vi "Init SVs.vi"(5 "error in":errorcluster) -> (19 "error out":errorcluster)   [LabVIEW 2015, in "cCRDS.lvclass"]
uses:
  cCRDS.lvclass
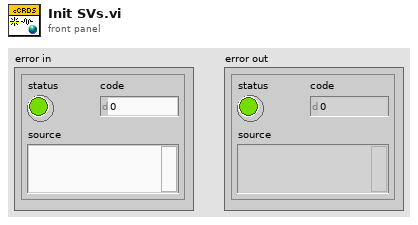
[diagram p1: front panel]
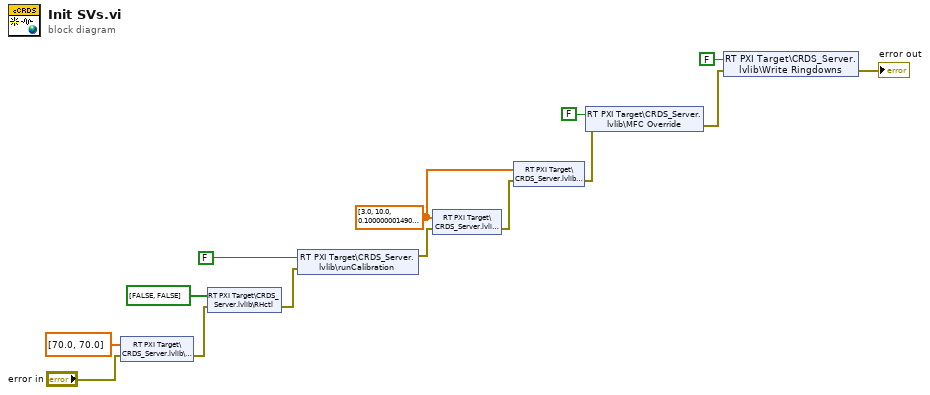
[diagram p0: block diagram]
diagram:
  w4 = sgl[] [3.0, 10.0, 0.1] ("Med")
  n1 = shared-variable "RT PXI Target\\CRDS_Server.lvlib\\RHsp"(sgl[] [70.0, 70.0] ("RHsp"), error in="error in") -> (error out=w13:errorcluster)
  n2 = shared-variable "RT PXI Target\\CRDS_Server.lvlib\\RHctl"(bool[] [FALSE, FALSE] ("RHctl"), error in=w13) -> (error out=w10:errorcluster)
  n3 = shared-variable "RT PXI Target\\CRDS_Server.lvlib\\runCalibration"(FALSE ("runCalibration"), error in=w10) -> (error out=w8:errorcluster)
  n4 = shared-variable "RT PXI Target\\CRDS_Server.lvlib\\Med"(w4, error in=w8) -> (error out=w5:errorcluster)
  n5 = shared-variable "RT PXI Target\\CRDS_Server.lvlib\\High"(w4, error in=w5) -> (error out=w6:errorcluster)
  n6 = shared-variable "RT PXI Target\\CRDS_Server.lvlib\\MFC Override"(FALSE ("MFC Override"), error in=w6) -> (error out=w2:errorcluster)
  n7 = shared-variable "RT PXI Target\\CRDS_Server.lvlib\\Write Ringdowns"(FALSE ("Write Ringdowns"), error in=w2) -> (error out=→"error out":errorcluster)
